vi "Do.vi"(8 "error in":errorcluster, 10 "Actor in":refnum<class "Actor.lvclass">, 11 "Enable Heater v MSG":refnum<class "Enable Heater MSG.lvclass">) -> (0 "error out":errorcluster, 2 "Actor out":refnum<class "Actor.lvclass">)   [LabVIEW 2017, in "Controller.lvlib" / "Enable Heater MSG.lvclass"]
doc: "(<B>Filename</B>: Actor Framework.lvlib:Message.lvclass:Do.vi)\n\nDefines what a message does when it is received by an actor. Generally, a message instructs an actor to invoke one of its methods. By default, this method does nothing. A child class must override it to define behavior. Create a child class by using the Actor Framework Message Maker dialog box."
uses:
  Enable Heater MSG.lvclass
  <vilib>/ActorFramework/Actor/Actor.lvclass
  Enable Heater MSG.lvclass/Enable Heater MSG.ctl
  gController.lvclass
  C:/Program Files (x86)/National Instruments/LabVIEW 2017/vi.lib/ActorFramework/Actor/Actor.lvclass
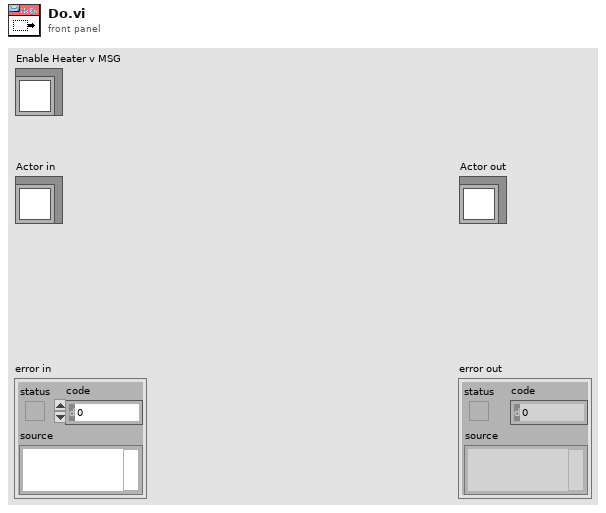
[diagram p1: front panel]
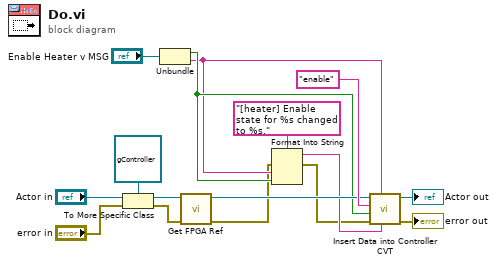
[diagram p0: block diagram]
diagram:
  n1 = To More Specific Class(target class=refnum<class "gController.lvclass"> refnum ("Controller.lvlib:gController"), reference="Actor in", error in="error in") -> (specific class reference=w7:refnum<class "gController.lvclass">, error out=w4:errorcluster)
  n2 = Unbundle("Enable Heater v MSG") -> (w11:bool, w10:string)
  n3 = call "Get FPGA Ref.vi"("error in (no error)"=w4, "Actor In"=w7) -> ("error out"=w2:errorcluster, "Actor Out"=w15:refnum<class "Actor.lvclass">)  [unwired: 7 in, 1 out]
  n4 = Format Into String(format string="[heater] Enable state for %s changed to %s.", error in=w2, w10, w11) -> (resulting string=w13:string, error out=w1:errorcluster)  [unwired: 1 in]
  n5 = call "Insert Data into Controller CVT.vi"("Update MSG"=w13, "Group"=w10, "error in"=w1, "Data"=w11, "tag"="enable", "Actor in"=w15) -> ("error out"=→"error out":errorcluster, "Actor Out"=→"Actor out":refnum<class "Actor.lvclass">)  [unwired: 4 in]
